vi "sequentialDataReader.vi"() -> ()   [LabVIEW 2012]
uses:
  ActiveMQBroker/ActiveMQBroker.lvclass
panel:
  out "Waveform Chart":dbl[](graph)
  in  "stopReader":bool
  in  "topic":string="testTopic"
  in  "port":string="61616"
  in  "host":string="localhost"
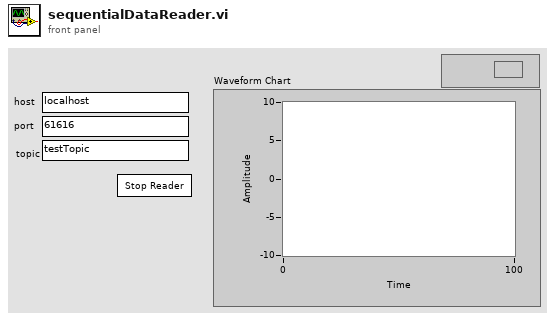
[diagram p1: front panel]
types:
  T1 = enum32{"invalid app kind", "Development System", "Run Time System", "Student Edition", "Embedded LabVIEW", "Evaluation", "Custom"}
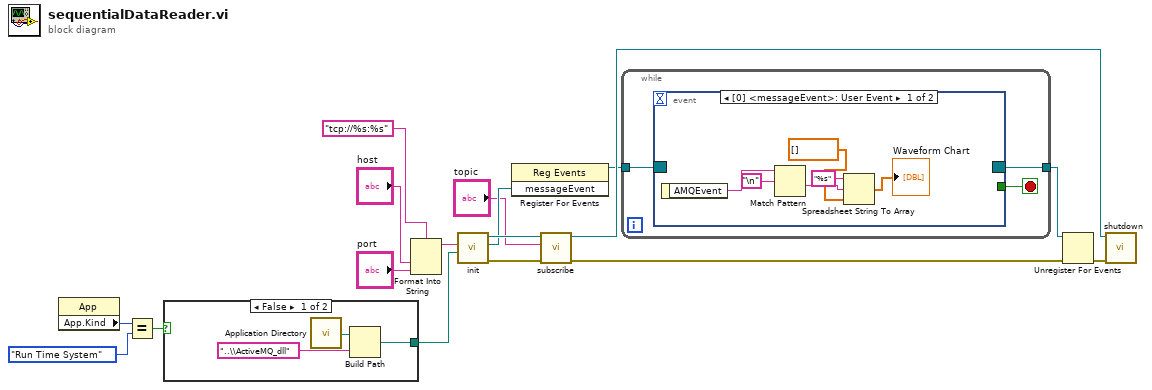
[diagram p0: block diagram]
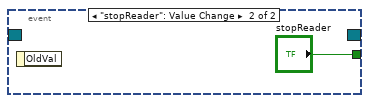
[diagram p2: hidden frame]
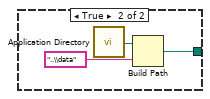
[diagram p3: hidden frame]
diagram:
  n1 = property class="App"() -> ("App.Kind"=w12:T1)  [unwired: 2 in, 2 out]
  n2 = Equal?(x=w12, y=T1."Run Time System") -> (x = y?=w10:bool)
  n3 = case shown="False" w10 {
    tunnel: [w18 w21] -> w17
    frame False {
      n4 = call <vilib>:"Application Directory.vi"() -> ("Application Directory"=w19:path)
      n5 = Build Path(base path=w19, name or relative path="..\\ActiveMQ_dll") -> (appended path=w18:path)
    }
    frame True {
      n6 = call <vilib>:"Application Directory.vi"() -> ("Application Directory"=w23:path)
      n7 = Build Path(base path=w23, name or relative path="..\\data") -> (appended path=w21:path)
    }
  }
  n8 = Format Into String(format string="tcp://%s:%s", "host", "port") -> (resulting string=w6:string)  [unwired: 2 in, 1 out]
  n9 = call "init.vi"("activeMQ_dll_directory"=w17, "brokerConnectionString"=w6) -> ("error out"=w16:errorcluster, "messageEvent"=w14:refnum<user-event>, "ActiveMQBroker out"=w15:refnum<class "ActiveMQBroker.lvclass">)  [unwired: 7 in]
  n10 = register-events(w14) -> (reference out=w5:refnum<event-registration>)  [unwired: 2 in, 1 out]
  n11 = call-dynamic "subscribe.vi"("error in (no error)"=w16, "source"="topic", "ActiveMQBroker in"=w15) -> ("error out"=w2:errorcluster, "ActiveMQBroker out"=w13:refnum<class "ActiveMQBroker.lvclass">)  [unwired: 7 in]
  n12 = while {
    tunnel: w5 -> [w26]
    tunnel: [w25] -> w4
    stop <- w24 stop-if-true
    n13 = event shown="[0] <messageEvent>: User Event" {
      selector: w26 -> [_ _]
      dyn-events: [_ _] -> w25
      timeout: _ -> [_ _]
      tunnel: [_ "stopReader"] -> w24
      event User Event {
        n14 = event-data() -> ("AMQEvent"=w32:string)  [unwired: 1 in]
        n15 = Match Pattern(string=w32, regular expression="\n") -> (after substring=w30:string)  [unwired: 1 in, 3 out]
        n16 = Spreadsheet String To Array(format string="%s", spreadsheet string=w30, array type (2D Dbl)=dbl[] [] ("anything")) -> (array=→"Waveform Chart":dbl[])  [unwired: 1 in]
      }
      event "stopReader": Value Change {
        n17 = event-data() -> ()  [unwired: 1 in, 1 out]
      }
    }
  }
  n18 = Unregister For Events(event registration refnum=w4, error in=w2) -> (error out=w3:errorcluster)
  n19 = call-dynamic "shutdown.vi"("error in (no error)"=w3, "ActiveMQBroker in"=w13) -> ()  [unwired: 8 in, 2 out]
